vi "SquidstatEventLoop.vi"(4 "AisUserEvents":T1 caption="SquidstatEvents", 5 "Device Name":string, 7 "error in (no error)":errorcluster) -> (3 "error out":errorcluster)   [LabVIEW 2018]
uses:
  SquidstatStructures/AisUserEvents.ctl
  private/VoidData.ctl
  private/Grounded.ctl
  private/ChannelExperimentNode.ctl
  SquidstatStructures/AisExperimentNode.ctl
  private/Channel.ctl
  private/ChannelDCData.ctl
  SquidstatStructures/AisDCData.ctl
  private/ChannelACData.ctl
  SquidstatStructures/AisACData.ctl
  SquidstatStructures/AisEvent_t.ctl
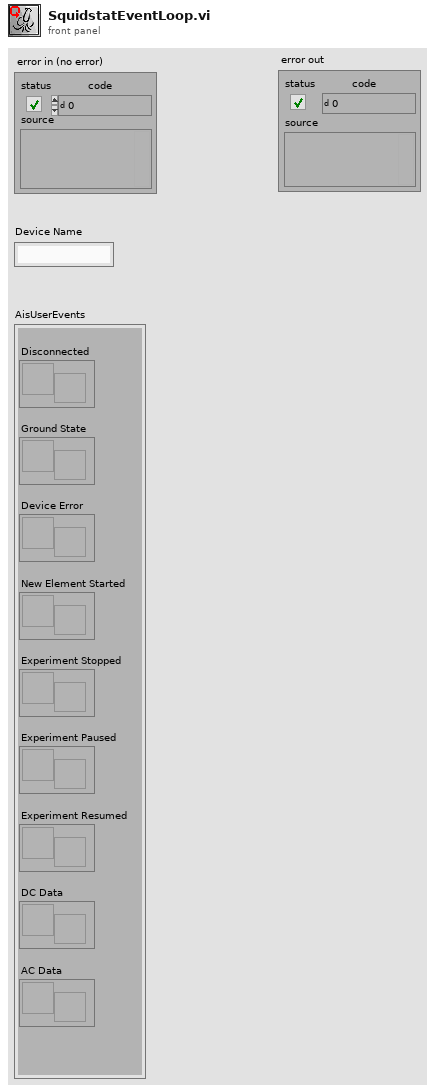
[diagram p1: front panel]
types:
  T1 = typedef "AisUserEvents.ctl" = cluster{"Disconnected":refnum<user-event>, "Ground State":refnum<user-event>, "Device Error":refnum<user-event>, "New Element Started":refnum<user-event>, "Experiment Stopped":refnum<user-event>, "Experiment Paused":refnum<user-event>, "Experiment Resumed":refnum<user-event>, "DC Data":refnum<user-event>, "AC Data":refnum<user-event>}
  T2 = typedef "AisEvent_t.ctl" = enum32{"AISEVENT_NULL", "AISEVENT_DISCONNECTED", "AISEVENT_GROUND_FLOAT_CHANGED", "AISEVENT_ERROR", "AISEVENT_ELEMENT_STARTED", "AISEVENT_EXP_STOPPED", "AISEVENT_PAUSED", "AISEVENT_RESUMED", "AISEVENT_DC_DATA", "AISEVENT_AC_DATA"}
  T3 = typedef "VoidData.ctl" = variant
  T4 = typedef "Grounded.ctl" = cluster{"Grounded":bool}
  T5 = typedef "ChannelExperimentNode.ctl" = cluster{"Channel":u8, "AisExperimentNode_c":T6}
  T6 = typedef "AisExperimentNode.ctl" = cluster{"Step Name":cluster{"char":u8, "char 2":u8, "char 3":u8, "char 4":u8, "char 5":u8, "char 6":u8, "char 7":u8, "char 8":u8, "char":u8, "char 9":u8, "char 10":u8, "char 11":u8, "char 12":u8, "char 13":u8, "char 14":u8, "char 15":u8, "char 16":u8, "char 17":u8, "char 18":u8, "char 19":u8, "char 20":u8, "char 21":u8, "char 22":u8, "char 23":u8, "char 24":u8, "char 25":u8, "char 26":u8, "char 27":u8, "char 28":u8, "char 29":u8, "char 30":u8, "char 31":u8, "char 32":u8, "char 33":u8, "char 34":u8, "char 35":u8, "char 36":u8, "char 37":u8, "char 38":u8, "char 39":u8, "char 40":u8, "char 41":u8, "char 42":u8, "char 43":u8, "char 44":u8, "char 45":u8, "char 46":u8, "char 47":u8, "char 48":u8, "char 49":u8, "char 50":u8, "char 50":u8}, "Step Number":i32, "Substep Number":i32, "Cycle Number":i32}
  T7 = typedef "Channel.ctl" = cluster{"Channel":dbl}
  T8 = typedef "AisDCData.ctl" = cluster{"timestamp":dbl, "workingElectrodeVoltage":dbl, "counterElectrodeVoltage":dbl, "current":dbl, "temperature":dbl}
  T9 = typedef "ChannelDCData.ctl" = cluster{"Channel":u8, "AisDCData":T8}
  T10 = typedef "AisACData.ctl" = cluster{"timestamp":dbl, "frequency":dbl, "absoluteImpedance":dbl, "realImpedance":dbl, "imagImpedance":dbl, "phaseAngle":dbl, "totalHarmonicDistortion":dbl, "numberOfCycles":dbl, "workingElectrodeDCVoltage":dbl, "DCCurrent":dbl, "currentAmplitude":dbl, "voltageAmplitude":dbl}
  T11 = typedef "ChannelACData.ctl" = cluster{"Channel":u8, "AisACData":T10}
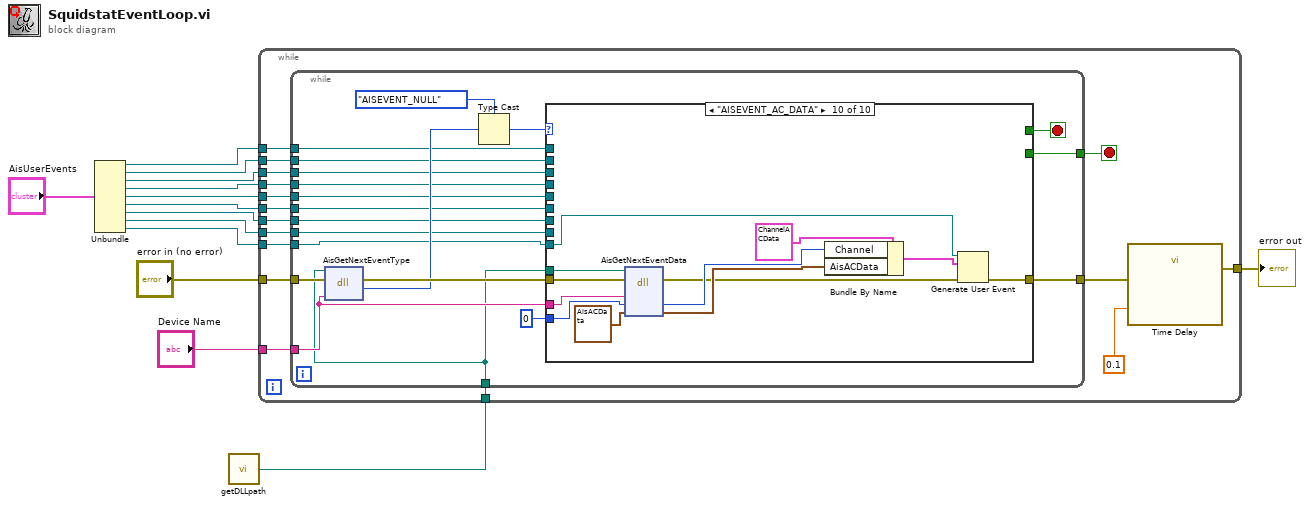
[diagram p0: block diagram]
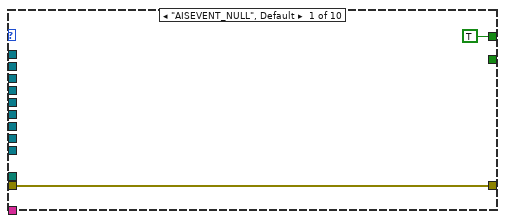
[diagram p2: hidden frame]
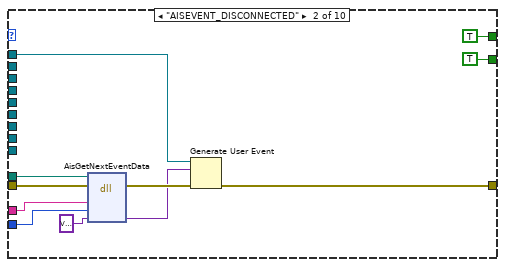
[diagram p3: hidden frame]
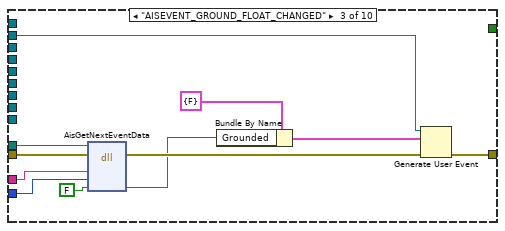
[diagram p4: hidden frame]
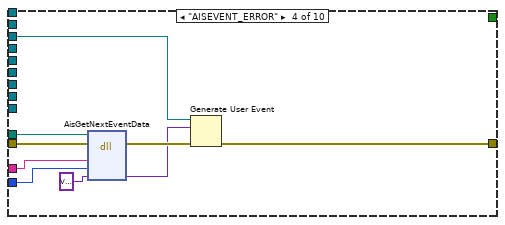
[diagram p5: hidden frame]
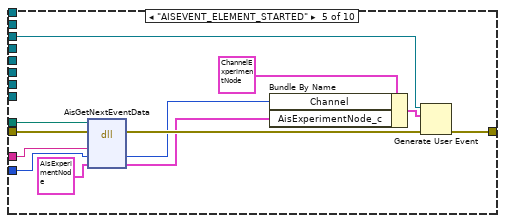
[diagram p6: hidden frame]
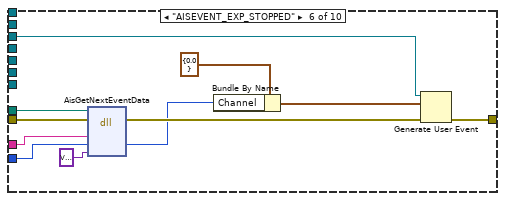
[diagram p7: hidden frame]
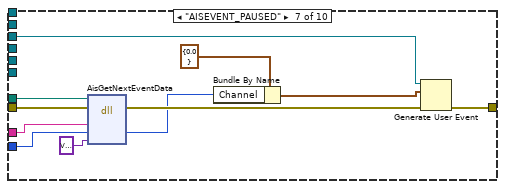
[diagram p8: hidden frame]
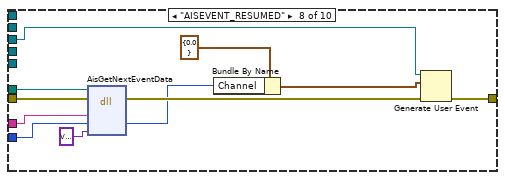
[diagram p9: hidden frame]
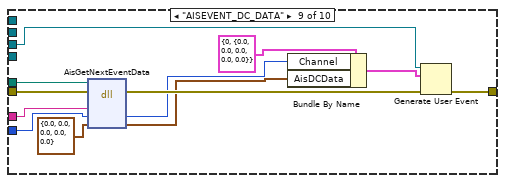
[diagram p10: hidden frame]
diagram:
  n1 = Unbundle("AisUserEvents") -> ("Disconnected"=w12:refnum<user-event>, "Ground State"=w11:refnum<user-event>, "Device Error"=w10:refnum<user-event>, "New Element Started"=w9:refnum<user-event>, "Experiment Stopped"=w8:refnum<user-event>, "Experiment Paused"=w7:refnum<user-event>, "Experiment Resumed"=w6:refnum<user-event>, "DC Data"=w5:refnum<user-event>, "AC Data"=w4:refnum<user-event>)
  n2 = call "getDLLpath.vi"() -> ("DLL_Path"=w1:path)
  n3 = while {
    tunnel: [w28] -> w2
    tunnel: "Device Name" -> [w30]
    tunnel: w12 -> [w27]
    tunnel: w11 -> [w26]
    tunnel: w10 -> [w25]
    tunnel: w9 -> [w24]
    tunnel: w8 -> [w23]
    tunnel: w7 -> [w22]
    tunnel: w6 -> [w21]
    tunnel: w5 -> [w20]
    tunnel: w4 -> [w19]
    tunnel: "error in (no error)" -> [w18]
    tunnel: w1 -> [w15]
    stop <- w17 stop-if-true
    n4 = while {
      tunnel: w30 -> [w47]
      tunnel: [w48] -> w29
      tunnel: w27 -> [w44]
      tunnel: w26 -> [w42]
      tunnel: w25 -> [w41]
      tunnel: w24 -> [w40]
      tunnel: w23 -> [w39]
      tunnel: w22 -> [w38]
      tunnel: w21 -> [w37]
      tunnel: w20 -> [w36]
      tunnel: w19 -> [w35]
      tunnel: w18 -> [w34]
      tunnel: [w32] -> w17
      tunnel: w15 -> [w31]
      stop <- w50 stop-if-true
      n5 = dll-call lib="?" fn="AisGetNextEventType" label="getNextEventType"(path in=w31, error in=w34, "DeviceName"=w47) -> (error out=w49:errorcluster, "Next Type"=w46:i32)  [unwired: 2 in, 1 out]
      n6 = Type Cast(type=AisEvent_t."AISEVENT_NULL" ("Enum"), x=w46) -> (*(type *) &x=w45:T2)
      n7 = case shown="\"AISEVENT_AC_DATA\"" w45 {
        tunnel: [TRUE TRUE _ _ _ _ _ _ _ _] -> w50
        tunnel: w49 -> [w51 w62 w74 w83 w94 w104 w117 w128 w139 w144]
        tunnel: [w51 w58 w69 w78 w87 w102 w113 w124 w137 w142] -> w48
        tunnel: w47 -> [_ w61 w73 w76 w95 w106 w115 w127 w140 w150]
        tunnel: w44 -> [_ w63 _ _ _ _ _ _ _ _]
        tunnel: u8 0 ("Channel") -> [_ w60 w72 w82 w90 w100 w111 w122 w131 w152]
        tunnel: w42 -> [_ _ w71 _ _ _ _ _ _ _]
        tunnel: w41 -> [_ _ _ w80 _ _ _ _ _ _]
        tunnel: w40 -> [_ _ _ _ w93 _ _ _ _ _]
        tunnel: w39 -> [_ _ _ _ _ w105 _ _ _ _]
        tunnel: w38 -> [_ _ _ _ _ _ w116 _ _ _]
        tunnel: w37 -> [_ _ _ _ _ _ _ w126 _ _]
        tunnel: w36 -> [_ _ _ _ _ _ _ _ w132 _]
        tunnel: w35 -> [_ _ _ _ _ _ _ _ _ w145]
        tunnel: [_ TRUE _ _ _ _ _ _ _ _] -> w32
        tunnel: w31 -> [_ w53 w64 w75 w84 w96 w107 w118 w129 w141]
        frame "AISEVENT_NULL", Default {
        }
        frame "AISEVENT_DISCONNECTED" {
          n8 = dll-call lib="?" fn="AisGetNextEventData" label="getNextEvent"(path in=w53, error in=w62, "deviceName"=w61, "channel"=w60, "eventOut"=T3 variant ("Void")) -> (error out=w59:errorcluster, "eventOut"=w56:T3)  [unwired: 4 in, 1 out]
          n9 = Generate User Event(user event=w63, event data cluster=w56, error in=w59) -> (error out=w58:errorcluster)  [unwired: 1 in, 1 out]
        }
        frame "AISEVENT_GROUND_FLOAT_CHANGED" {
          n10 = dll-call lib="?" fn="AisGetNextEventData" label="getNextEvent"(path in=w64, error in=w74, "deviceName"=w73, "channelOut"=w72, "eventOut"=FALSE) -> (error out=w70:errorcluster, "eventOut"=w66:bool)  [unwired: 4 in, 1 out]
          n11 = Bundle By Name(cluster=T4 {"Grounded"=FALSE} ("Grounded"), "Grounded"=w66) -> (w65:T4)
          n12 = Generate User Event(user event=w71, event data cluster=w65, error in=w70) -> (error out=w69:errorcluster)  [unwired: 1 in, 1 out]
        }
        frame "AISEVENT_ERROR" {
          n13 = dll-call lib="?" fn="AisGetNextEventData" label="getNextEvent"(path in=w75, error in=w83, "deviceName"=w76, "channelOut"=w82, "eventOut"=T3 variant ("Void")) -> (error out=w79:errorcluster, "eventOut"=w77:T3)  [unwired: 4 in, 1 out]
          n14 = Generate User Event(user event=w80, event data cluster=w77, error in=w79) -> (error out=w78:errorcluster)  [unwired: 1 in, 1 out]
        }
        frame "AISEVENT_ELEMENT_STARTED" {
          n15 = dll-call lib="?" fn="AisGetNextEventData" label="getNextEvent"(path in=w84, error in=w94, "deviceName"=w95, "channelOut"=w90, "eventOut"=T6 {"Step Name"={"char"=0, "char 2"=0, "char 3"=0, "char 4"=0, "char 5"=0, "char 6"=0, "char 7"=0, "char 8"=0, "char"=0, "char 9"=0, "char 10"=0, "char 11"=0, "char 12"=0, "char 13"=0, "char 14"=0, "char 15"=0, "char 16"=0, "char 17"=0, "char 18"=0, "char 19"=0, "char 20"=0, "char 21"=0, "char 22"=0, "char 23"=0, "char 24"=0, "char 25"=0, "char 26"=0, "char 27"=0, "char 28"=0, "char 29"=0, "char 30"=0, "char 31"=0, "char 32"=0, "char 33"=0, "char 34"=0, "char 35"=0, "char 36"=0, "char 37"=0, "char 38"=0, "char 39"=0, "char 40"=0, "char 41"=0, "char 42"=0, "char 43"=0, "char 44"=0, "char 45"=0, "char 46"=0, "char 47"=0, "char 48"=0, "char 49"=0, "char 50"=0, "char 50"=0}, "Step Number"=0, "Substep Number"=0, "Cycle Number"=0} ("AisExperimentNode_c")) -> (error out=w88:errorcluster, "channelOut"=w86:u8, "eventOut"=w85:T6)  [unwired: 3 in, 1 out]
          n16 = Bundle By Name(cluster=T5 {"Channel"=0, "AisExperimentNode_c"={"Step Name"={"char"=0, "char 2"=0, "char 3"=0, "char 4"=0, "char 5"=0, "char 6"=0, "char 7"=0, "char 8"=0, "char"=0, "char 9"=0, "char 10"=0, "char 11"=0, "char 12"=0, "char 13"=0, "char 14"=0, "char 15"=0, "char 16"=0, "char 17"=0, "char 18"=0, "char 19"=0, "char 20"=0, "char 21"=0, "char 22"=0, "char 23"=0, "char 24"=0, "char 25"=0, "char 26"=0, "char 27"=0, "char 28"=0, "char 29"=0, "char 30"=0, "char 31"=0, "char 32"=0, "char 33"=0, "char 34"=0, "char 35"=0, "char 36"=0, "char 37"=0, "char 38"=0, "char 39"=0, "char 40"=0, "char 41"=0, "char 42"=0, "char 43"=0, "char 44"=0, "char 45"=0, "char 46"=0, "char 47"=0, "char 48"=0, "char 49"=0, "char 50"=0, "char 50"=0}, "Step Number"=0, "Substep Number"=0, "Cycle Number"=0}} ("ChannelExperimentNode"), "Channel"=w86, "AisExperimentNode_c"=w85) -> (w89:T5)
          n17 = Generate User Event(user event=w93, event data cluster=w89, error in=w88) -> (error out=w87:errorcluster)  [unwired: 1 in, 1 out]
        }
        frame "AISEVENT_EXP_STOPPED" {
          n18 = dll-call lib="?" fn="AisGetNextEventData" label="getNextEvent"(path in=w96, error in=w104, "deviceName"=w106, "channelOut"=w100, "eventOut"=T3 variant ("Void")) -> (error out=w103:errorcluster, "channelOut"=w98:u8)  [unwired: 4 in, 1 out]
          n19 = Bundle By Name(cluster=T7 {"Channel"=0.0} ("Channel"), "Channel"=w98) -> (w97:T7)
          n20 = Generate User Event(user event=w105, event data cluster=w97, error in=w103) -> (error out=w102:errorcluster)  [unwired: 1 in, 1 out]
        }
        frame "AISEVENT_PAUSED" {
          n21 = dll-call lib="?" fn="AisGetNextEventData" label="getNextEvent"(path in=w107, error in=w117, "deviceName"=w115, "channelOut"=w111, "eventOut"=T3 variant ("Void")) -> (error out=w114:errorcluster, "channelOut"=w110:u8)  [unwired: 4 in, 1 out]
          n22 = Bundle By Name(cluster=T7 {"Channel"=0.0} ("Channel"), "Channel"=w110) -> (w108:T7)
          n23 = Generate User Event(user event=w116, event data cluster=w108, error in=w114) -> (error out=w113:errorcluster)  [unwired: 1 in, 1 out]
        }
        frame "AISEVENT_RESUMED" {
          n24 = dll-call lib="?" fn="AisGetNextEventData" label="getNextEvent"(path in=w118, error in=w128, "deviceName"=w127, "channelOut"=w122, "eventOut"=T3 variant ("Void")) -> (error out=w125:errorcluster, "channelOut"=w120:u8)  [unwired: 4 in, 1 out]
          n25 = Bundle By Name(cluster=T7 {"Channel"=0.0} ("Channel"), "Channel"=w120) -> (w119:T7)
          n26 = Generate User Event(user event=w126, event data cluster=w119, error in=w125) -> (error out=w124:errorcluster)  [unwired: 1 in, 1 out]
        }
        frame "AISEVENT_DC_DATA" {
          n27 = dll-call lib="?" fn="AisGetNextEventData" label="getNextEvent"(path in=w129, error in=w139, "deviceName"=w140, "channelOut"=w131, "eventOut"=T8 {"timestamp"=0.0, "workingElectrodeVoltage"=0.0, "counterElectrodeVoltage"=0.0, "current"=0.0, "temperature"=0.0} ("AisDCData")) -> (error out=w138:errorcluster, "channelOut"=w130:u8, "eventOut"=w134:T8)  [unwired: 3 in, 1 out]
          n28 = Bundle By Name(cluster=T9 {"Channel"=0, "AisDCData"={"timestamp"=0.0, "workingElectrodeVoltage"=0.0, "counterElectrodeVoltage"=0.0, "current"=0.0, "temperature"=0.0}} ("ChannelDCData"), "Channel"=w130, "AisDCData"=w134) -> (w133:T9)
          n29 = Generate User Event(user event=w132, event data cluster=w133, error in=w138) -> (error out=w137:errorcluster)  [unwired: 1 in, 1 out]
        }
        frame "AISEVENT_AC_DATA" {
          n30 = dll-call lib="?" fn="AisGetNextEventData" label="getNextEvent"(path in=w141, error in=w144, "deviceName"=w150, "channelOut"=w152, "eventOut"=T10 {"timestamp"=0.0, "frequency"=0.0, "absoluteImpedance"=0.0, "realImpedance"=0.0, "imagImpedance"=0.0, "phaseAngle"=0.0, "totalHarmonicDistortion"=0.0, "numberOfCycles"=0.0, "workingElectrodeDCVoltage"=0.0, "DCCurrent"=0.0, "currentAmplitude"=0.0, "voltageAmplitude"=0.0} ("AisACData")) -> (error out=w143:errorcluster, "channelOut"=w149:u8, "eventOut"=w147:T10)  [unwired: 3 in, 1 out]
          n31 = Bundle By Name(cluster=T11 {"Channel"=0, "AisACData"={"timestamp"=0.0, "frequency"=0.0, "absoluteImpedance"=0.0, "realImpedance"=0.0, "imagImpedance"=0.0, "phaseAngle"=0.0, "totalHarmonicDistortion"=0.0, "numberOfCycles"=0.0, "workingElectrodeDCVoltage"=0.0, "DCCurrent"=0.0, "currentAmplitude"=0.0, "voltageAmplitude"=0.0}} ("ChannelACData"), "Channel"=w149, "AisACData"=w147) -> (w146:T11)
          n32 = Generate User Event(user event=w145, event data cluster=w146, error in=w143) -> (error out=w142:errorcluster)  [unwired: 1 in, 1 out]
        }
      }
    }
    n33 = call "Time Delay"("error in (no error)"=w29, "Delay Time (s)"=0.1) -> ("error out"=w28:errorcluster)  [unwired: 9 in]
  }
  "error out" <- w2
